vi "RegisterPubSub.vi"(2 "LogPath in":path, 3 "New server ROS":T2) -> (0 "LogPath out":path, 1 "MyState":T1)   [LabVIEW 2014]
doc: "Registers a publisher or subscriber with the master and returns the state"
uses:
  _ROSControl.ctl
  _ROSDirection.ctl
  Console/Servers/ServerSubs/MyState.ctl
  _ROSDefinition.vi
panel:
  out "Response":T4
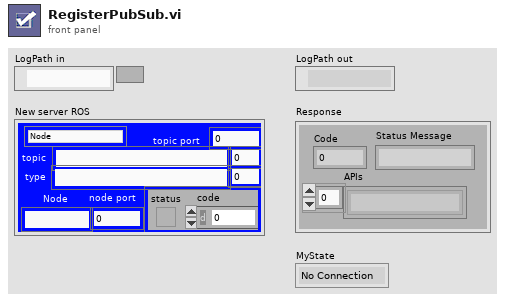
[diagram p1: front panel]
types:
  T1 = typedef "MyState.ctl" = enum16{"No Connection", "Registered", "Connected", "Close"}
  T2 = typedef "_ROSControl.ctl" = cluster{"topic port":u16, "Node":string, "topic":string, "type":string, "node port":u16, "error ":errorcluster, "Direction":T3, "Update (ms)":u16, "FIFO size":u16}
  T3 = typedef "_ROSDirection.ctl" = enum16{"Node", "Publisher", "Subscriber", "ServiceClient", "ServiceProvider"}
  T4 = cluster{"Code":i32, "Status Message":string, "APIs":string[]}
  T5 = enum16{"Reset Log", "Add Client", "Remove Client", "Add Task"}
  T6 = enum16{"http://IP:port", "http://IP", "IP:port", "IP only"}
  T7 = typedef "ROSLog.ctl" = cluster{"Sent":string, "Reply":string, "MethodName":string, "success":bool, "Dir1":string, "Dir2":string, "Time Stamp":string, "error":errorcluster, "Preamble":string, "Midamble":string, "Postamble":string}
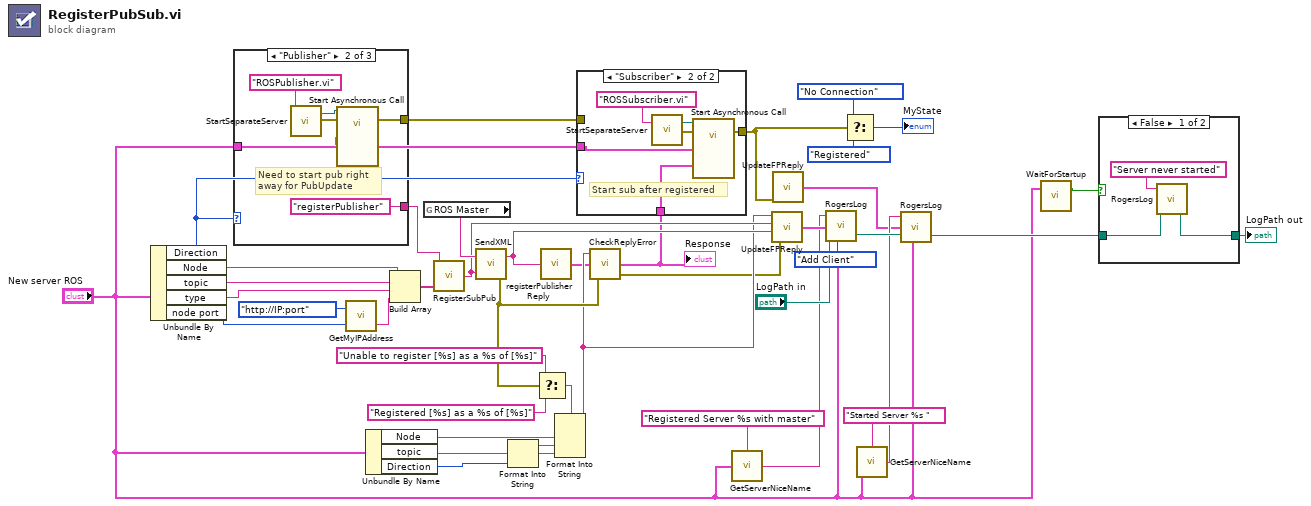
[diagram p0: block diagram]
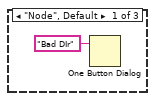
[diagram p4: hidden frame]
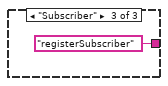
[diagram p5: hidden frame]
diagram:
  n1 = Unbundle By Name("New server ROS") -> ("Direction"=w7:T3, "Node"=w35:string, "topic"=w34:string, "type"=w33:string, "node port"=w32:u16)
  n2 = case shown="\"Publisher\"" w7 {
    tunnel: [_ "registerPublisher" ("MethodName") "registerSubscriber" ("MethodName")] -> w40
    tunnel: [_ w44 _] -> w5
    tunnel: "New server ROS" -> [_ w43 _]
    frame "Node", Default {
      n3 = One Button Dialog(message="Bad DIr") -> ()  [unwired: 1 in, 1 out]
    }
    frame "Publisher" {
      # "Need to start pub right\naway for PubUpdate"
      n4 = call "StartSeparateServer.vi"("Server"="ROSPublisher.vi" ("name (unnamed)")) -> ("error out"=w46:errorcluster, "Ref out"=w47:refnum<vi>)  [unwired: 1 in]
      n5 = call-by-ref "Start Asynchronous Call"(reference=w47, error in=w46, "ROS"=w43) -> (error out=w44:errorcluster)  [unwired: 3 in, 1 out]
    }
    frame "Subscriber" {
    }
  }
  n6 = call "GetMyIPAddress.vi"("Port"=w32, "Format"=T6."http://IP:port") -> ("URI"=w31:string)  [unwired: 1 out]
  n7 = Unbundle By Name("New server ROS") -> ("Node"=w25:string, "topic"=w26:string, "Direction"=w24:T3)
  n8 = Build Array(w35, w34, w33, w31) -> (w36:string[])
  n9 = global read "_ROSDefinition.vi" "ROS Master"() -> (w37:string)
  n10 = call "RegisterSubPub.vi"("Parameters"=w36, "MethodName"=w40) -> ("XML"=w29:string)
  n11 = call "SendXML.vi"("Send"=w29, "URI in"=w37) -> ("error out"=w22:errorcluster, "Reply"=w28:string)
  n12 = Format Into String(w24) -> (resulting string=w23:string)  [unwired: 3 in, 1 out]
  n13 = Select(t="Unable to register [%s] as a %s of [%s]" ("format string"), s=w22, f="Registered [%s] as a %s of [%s]" ("format string")) -> (s? t:f=w19:string)
  n14 = call "registerPublisherReply.vi"("Response"=w28) -> ("Response"=w8:T4)
  "Response" <- w8
  n15 = Format Into String(format string=w19, w25, w23, w26) -> (resulting string=w18:string)  [unwired: 2 in, 1 out]
  n16 = case shown="\"Subscriber\"" w7 {
    tunnel: w8 -> [_ w51]
    tunnel: "New server ROS" -> [_ w52]
    tunnel: [w50 w53] -> w6
    tunnel: w5 -> [w50 _]
    frame Default {
    }
    frame "Subscriber" {
      # "Start sub after registered"
      n17 = call "StartSeparateServer.vi"("Server"="ROSSubscriber.vi" ("name (unnamed)")) -> ("error out"=w55:errorcluster, "Ref out"=w56:refnum<vi>)  [unwired: 1 in]
      n18 = call-by-ref "Start Asynchronous Call"(reference=w56, error in=w55, "Response"=w51, "ROS"=w52) -> (error out=w53:errorcluster)  [unwired: 2 in, 1 out]
    }
  }
  n19 = call "CheckReplyError.vi"("error in"=w22, "Response"=w8, "Error String"=w18) -> ("error out"=w11:errorcluster)  [unwired: 2 out]
  n20 = call "GetServerNiceName.vi"("ROS"="New server ROS", "Text to add"="Registered Server %s with master") -> ("String"=w15:string)
  n21 = call "UpdateFPReply.vi"("error in (no error)"=w11, "Reply"=w28, "Sent"=w29, "method"=w18) -> ("Log"=w27:T7)
  n22 = call "UpdateFPReply.vi"("error in (no error)"=w6) -> ("Log"=w12:T7)  [unwired: 3 in]
  n23 = call "RogersLog.vi"("Text to add"=w15, "ROS"="New server ROS", "Log"=w27, "LogPath in"="LogPath in", "Task"=T5."Add Client") -> ("LogPath out"=w17:path)  [unwired: 1 out]
  n24 = Select(t=MyState."No Connection" ("MyState"), s=w6, f=MyState."Registered" ("MyState")) -> (s? t:f=→"MyState":T1)
  n25 = call "GetServerNiceName.vi"("ROS"="New server ROS", "Text to add"="Started Server %s ") -> ("String"=w13:string)
  n26 = call "RogersLog.vi"("Text to add"=w13, "ROS"="New server ROS", "Log"=w12, "LogPath in"=w17) -> ("LogPath out"=w4:path)  [unwired: 1 in, 1 out]
  n27 = call "WaitForStartup.vi"("ROS"="New server ROS") -> ("success?"=w1:bool)  [unwired: 2 in]
  n28 = case shown="False" w1 {
    tunnel: w4 -> [w58 w60]
    tunnel: [w57 w60] -> w3
    frame False {
      n29 = call "RogersLog.vi"("Text to add"="Server never started", "LogPath in"=w58) -> ("LogPath out"=w57:path)  [unwired: 3 in, 1 out]
    }
    frame True {
    }
  }
  "LogPath out" <- w3
